vi "例程23-数据记录文件的创建.vi"() -> ()   [LabVIEW 2016]
panel:
  out "记录":cluster{"温度":dbl, "日期":string, "时间":string}
  in  "温度计":dbl(slide) scale=0.0..100.0
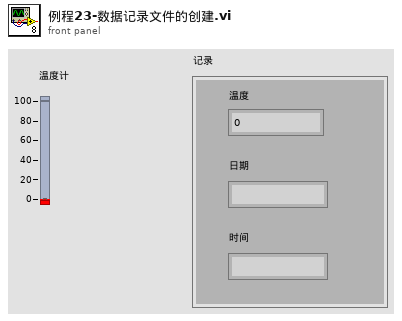
[diagram p1: front panel]
types:
  T1 = enum16{"open", "replace", "create", "open or create", "replace or create", "replace or create with confirmation"}
  T2 = cluster{"温度计":dbl, "date string":string, "time string":string}
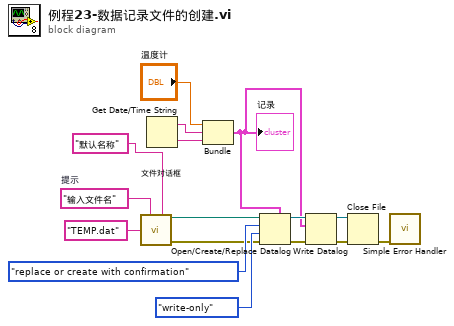
[diagram p0: block diagram]
diagram:
  w15 = "输入文件名"  # 提示
  n1 = call "文件对话框"("prompt"=w15, "button label"="默认名称", "default name"="TEMP.dat") -> ("selected path"=w12:path, "error out"=w1:errorcluster)  [unwired: 9 in, 2 out]
  n2 = Get Date/Time String() -> (date string=w6:string, time string=w5:string)  [unwired: 3 in]
  n3 = Bundle("温度计"="温度计", "date string"=w6, "time string"=w5) -> (w4:T2)  [unwired: 1 in]
  "记录" <- w4
  n4 = Open/Create/Replace Datalog(5:w4, 8:w1, 9:enum16{"read/write", "read-only", "write-only"}."write-only" ("权限(0:read/write)"), 10:T1."replace or create with confirmation" ("操作(0:open)"), 11:w12) -> (0:w8:errorcluster, 3:w9:refnum<k1>)  [unwired: 1 in, 1 out]
  n5 = Write Datalog(4:w8, 6:w4, 7:w9) -> (0:w3:errorcluster, 3:w2:refnum<k1>)
  n6 = Close File(refnum=w2, error in=w3) -> (error out=w16:errorcluster)  [unwired: 1 out]
  n7 = call <vilib>:"Simple Error Handler.vi"("error in (no error)"=w16) -> ()  [unwired: 4 in, 5 out]
